vi "SUB-BLE Rx data (Debug)-CDC.vi"(8 "data in":u8[](array[numeric]) format="%2x") -> (2 "CDC debug":T1 caption="CDC Debugging data" {"Right Wing-C, C6/C0" format="%#.9f"; "Right Wing-B, C5/C0" format="%#.9f"; "Right Wing-A, C4/C0" format="%#.9f"; "Left Wing-C, C3/C0" format="%#.9f"; "Left Wing-B, C2/C0" format="%#.9f"; "Left Wing-A, C1/C0" format="%#.9f"}, 3 "CDC mon":T1 caption="CDC Monitoring data" {"Right Wing-C, C6/C0" format="%#.9f"; "Right Wing-B, C5/C0" format="%#.9f"; "Right Wing-A, C4/C0" format="%#.9f"; "Left Wing-C, C3/C0" format="%#.9f"; "Left Wing-B, C2/C0" format="%#.9f"; "Left Wing-A, C1/C0" format="%#.9f"})   [LabVIEW 2015]
doc: "Use this template to create an application that executes repeatedly until you click the Stop button. This template polls the state of the Stop button and does not use events. Use the Top-Level Application template (not available in the Base package) to create a single-loop application with event handling."
panel:
  out "BLE Packet (buf)":u8[](array[numeric])
  out "BLE Packet (data)":u8[](array[numeric])
  # "BLE 수신 데이터를 처리: Debugging data"
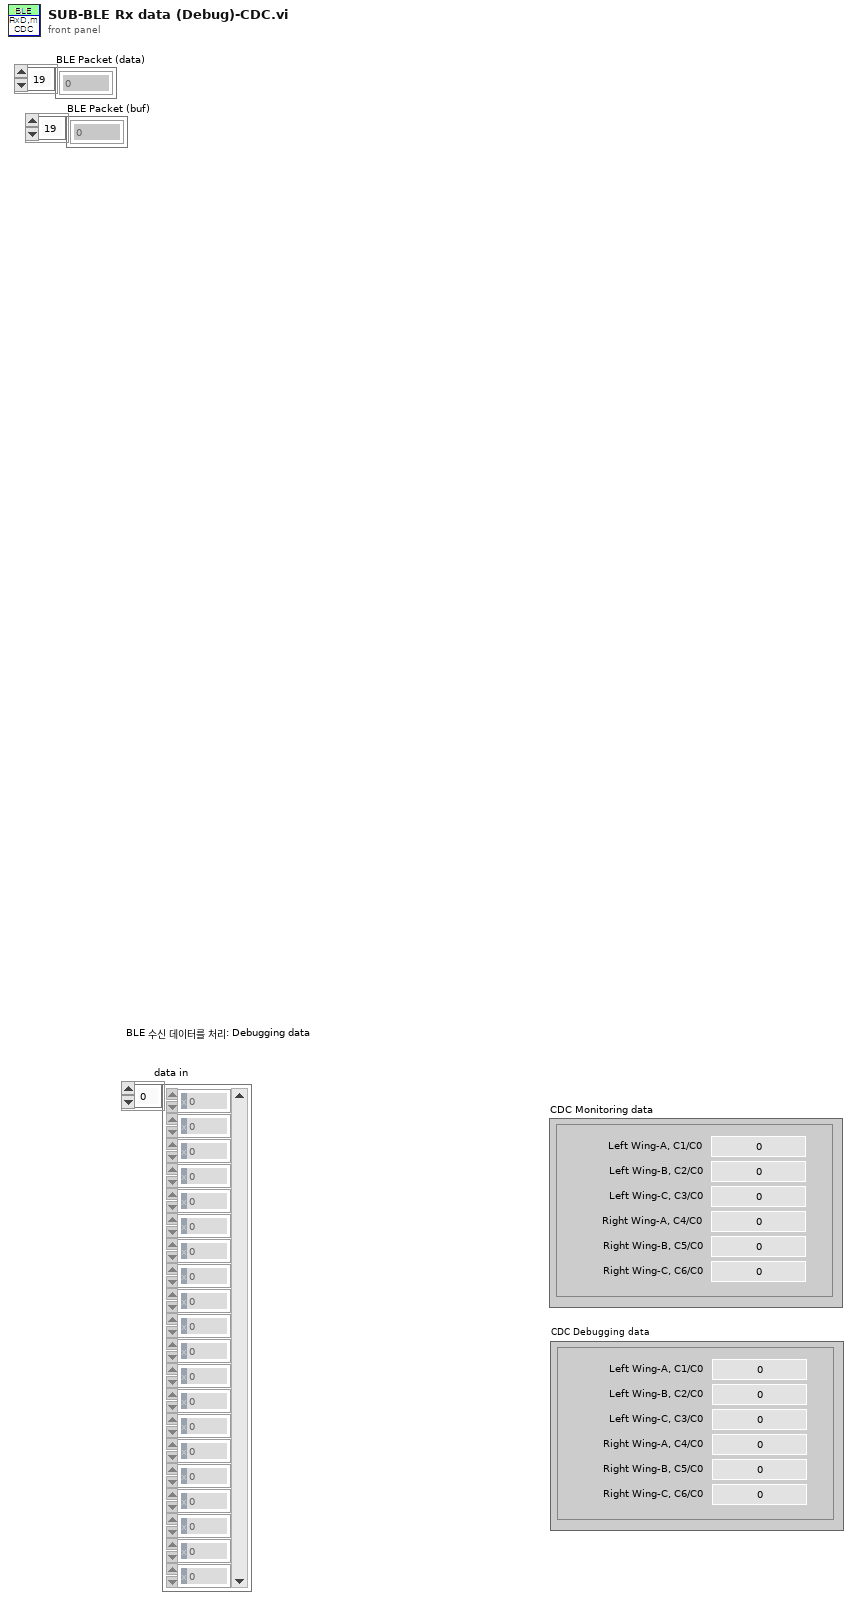
[diagram p1: front panel]
types:
  T1 = typedef "컨트롤-CDC data.ctl" = cluster{"Left Wing-A, C1/C0":dbl, "Left Wing-B, C2/C0":dbl, "Left Wing-C, C3/C0":dbl, "Right Wing-A, C4/C0":dbl, "Right Wing-B, C5/C0":dbl, "Right Wing-C, C6/C0":dbl}
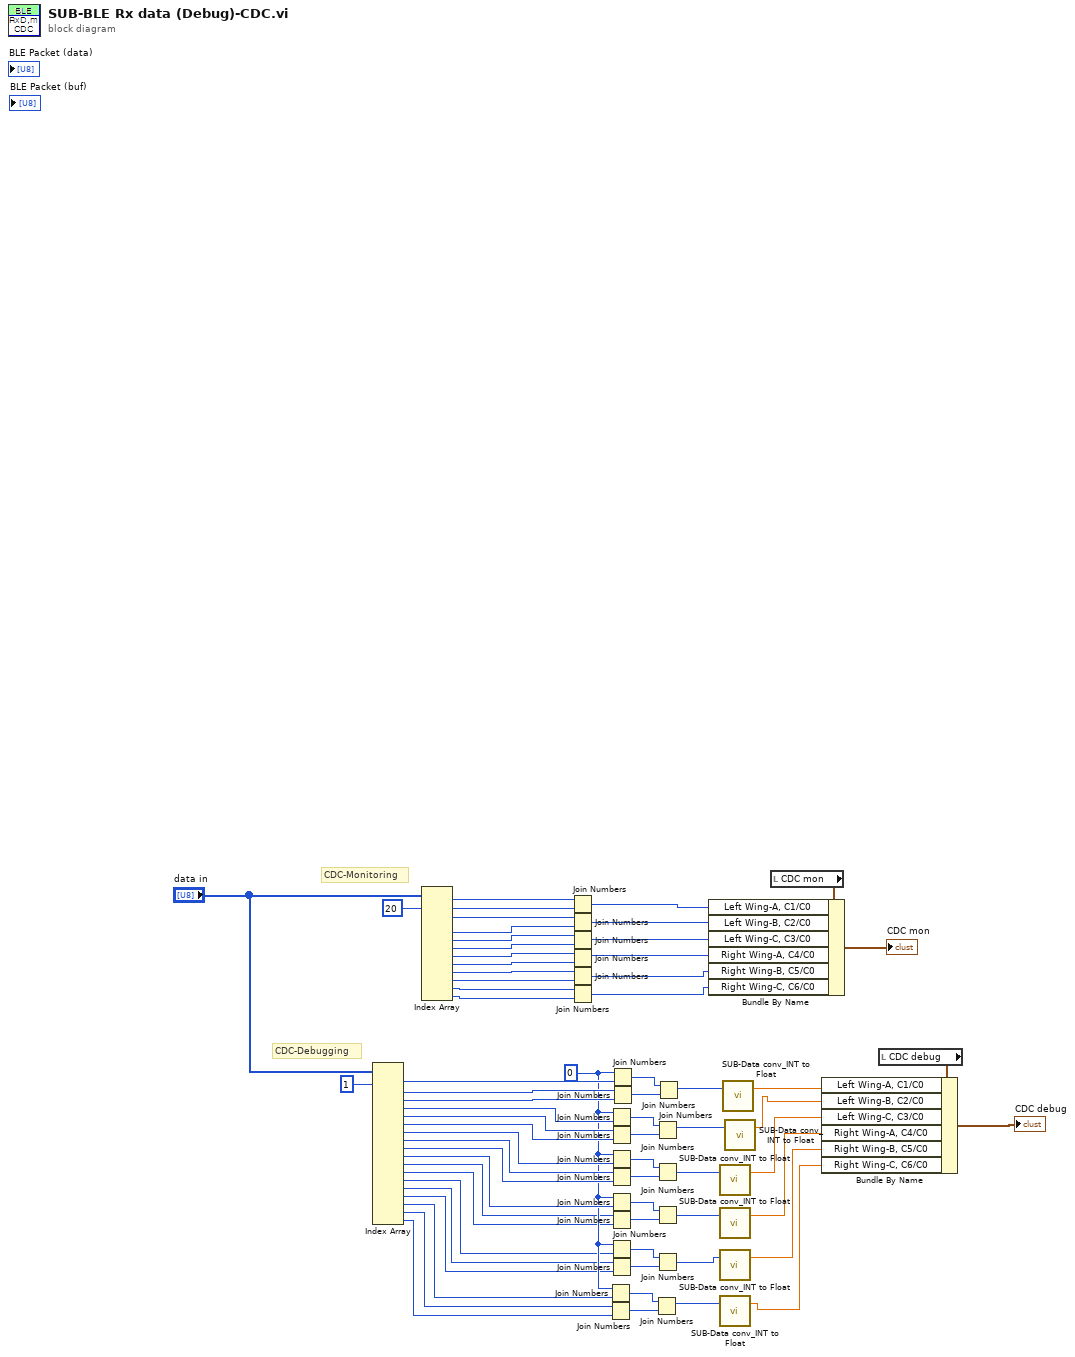
[diagram p0: block diagram]
diagram:
  w21 = u8 0 ("hi")
  # "CDC-Debugging"
  # "CDC-Monitoring"
  n1 = Index Array(array="data in", index #1=1 ("인덱스")) -> (element #1=w43:u8, element #2=w42:u8, element #3=w41:u8, element #4=w28:u8, element #5=w27:u8, element #6=w26:u8, element #7=w25:u8, element #8=w24:u8, element #9=w23:u8, element #10=w22:u8, element #11=w20:u8, element #12=w19:u8, element #13=w18:u8, element #14=w17:u8, element #15=w16:u8, element #16=w15:u8, element #17=w14:u8, element #18=w13:u8)  [unwired: 17 in]
  n2 = Index Array(array="data in", index #1=20 ("인덱스")) -> (element #1=w66:u8, element #2=w65:u8, element #3=w64:u8, element #4=w63:u8, element #5=w62:u8, element #6=w61:u8, element #7=w60:u8, element #8=w59:u8, element #9=w58:u8, element #10=w57:u8, element #11=w56:u8, element #12=w55:u8)  [unwired: 11 in]
  n3 = Join Numbers(hi=w66, lo=w65) -> ((hi.lo)=w53:u16)
  n4 = Join Numbers(hi=w64, lo=w63) -> ((hi.lo)=w52:u16)
  n5 = Join Numbers(hi=w62, lo=w61) -> ((hi.lo)=w51:u16)
  n6 = Join Numbers(hi=w60, lo=w59) -> ((hi.lo)=w50:u16)
  n7 = Join Numbers(hi=w58, lo=w57) -> ((hi.lo)=w49:u16)
  n8 = Join Numbers(hi=w56, lo=w55) -> ((hi.lo)=w48:u16)
  n9 = Join Numbers(hi=w21, lo=w15) -> ((hi.lo)=w30:u16)
  n10 = Join Numbers(hi=w14, lo=w13) -> ((hi.lo)=w29:u16)
  n11 = Join Numbers(hi=w21, lo=w28) -> ((hi.lo)=w38:u16)
  n12 = Join Numbers(hi=w27, lo=w26) -> ((hi.lo)=w37:u16)
  n13 = Join Numbers(hi=w21, lo=w25) -> ((hi.lo)=w35:u16)
  n14 = Join Numbers(hi=w24, lo=w23) -> ((hi.lo)=w36:u16)
  n15 = Join Numbers(hi=w21, lo=w22) -> ((hi.lo)=w34:u16)
  n16 = Join Numbers(hi=w20, lo=w19) -> ((hi.lo)=w33:u16)
  n17 = Join Numbers(hi=w21, lo=w18) -> ((hi.lo)=w31:u16)
  n18 = Join Numbers(hi=w17, lo=w16) -> ((hi.lo)=w32:u16)
  n19 = Join Numbers(hi=w21, lo=w43) -> ((hi.lo)=w39:u16)
  n20 = Join Numbers(hi=w42, lo=w41) -> ((hi.lo)=w40:u16)
  n21 = Join Numbers(hi=w30, lo=w29) -> ((hi.lo)=w11:u32)
  n22 = Join Numbers(hi=w38, lo=w37) -> ((hi.lo)=w8:u32)
  n23 = Join Numbers(hi=w35, lo=w36) -> ((hi.lo)=w9:u32)
  n24 = Join Numbers(hi=w34, lo=w33) -> ((hi.lo)=w10:u32)
  n25 = Join Numbers(hi=w31, lo=w32) -> ((hi.lo)=w12:u32)
  n26 = Join Numbers(hi=w39, lo=w40) -> ((hi.lo)=w7:u32)
  n27 = call "SUB-Data conv_INT to Float.vi"("U32"=w9) -> ("FP32"=w4:sgl)  [unwired: 2 in]
  n28 = call "SUB-Data conv_INT to Float.vi"("U32"=w10) -> ("FP32"=w3:sgl)  [unwired: 2 in]
  n29 = call "SUB-Data conv_INT to Float.vi"("U32"=w12) -> ("FP32"=w2:sgl)  [unwired: 2 in]
  n30 = call "SUB-Data conv_INT to Float.vi"("U32"=w11) -> ("FP32"=w1:sgl)  [unwired: 2 in]
  n31 = call "SUB-Data conv_INT to Float.vi"("U32"=w7) -> ("FP32"=w6:sgl)  [unwired: 2 in]
  n32 = call "SUB-Data conv_INT to Float.vi"("U32"=w8) -> ("FP32"=w5:sgl)  [unwired: 2 in]
  n33 = local read "CDC mon"() -> (w68:T1)
  n34 = Bundle By Name(cluster=w68, "Left Wing-A, C1/C0"=w53, "Left Wing-B, C2/C0"=w52, "Left Wing-C, C3/C0"=w51, "Right Wing-A, C4/C0"=w50, "Right Wing-B, C5/C0"=w49, "Right Wing-C, C6/C0"=w48) -> (→"CDC mon":T1)
  n35 = local read "CDC debug"() -> (w46:T1)
  n36 = Bundle By Name(cluster=w46, "Left Wing-A, C1/C0"=w6, "Left Wing-B, C2/C0"=w5, "Left Wing-C, C3/C0"=w4, "Right Wing-A, C4/C0"=w3, "Right Wing-B, C5/C0"=w2, "Right Wing-C, C6/C0"=w1) -> (→"CDC debug":T1)
